vi "Lecture ParamStack.vi"(8 "errin":errorcluster, 11 "varriante":string) -> (0 "error out":errorcluster caption="errout")   [LabVIEW 2020]
uses:
  <vilib>/Utility/config.llb/Read Key (Double).vi
  <vilib>/Utility/config.llb/Read Key (String).vi
  Param_Stack.vi
  <vilib>/Utility/config.llb/NI_LVConfig.lvlib
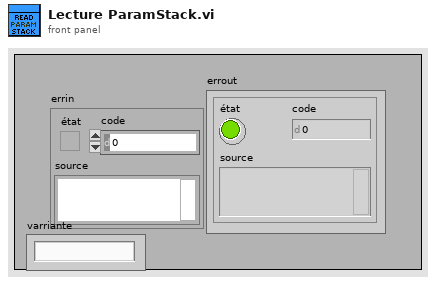
[diagram p1: front panel]
types:
  T1 = typedef "NI_LVConfig.lvlib/Config Data RefNum.ctl" = refnum<k1>
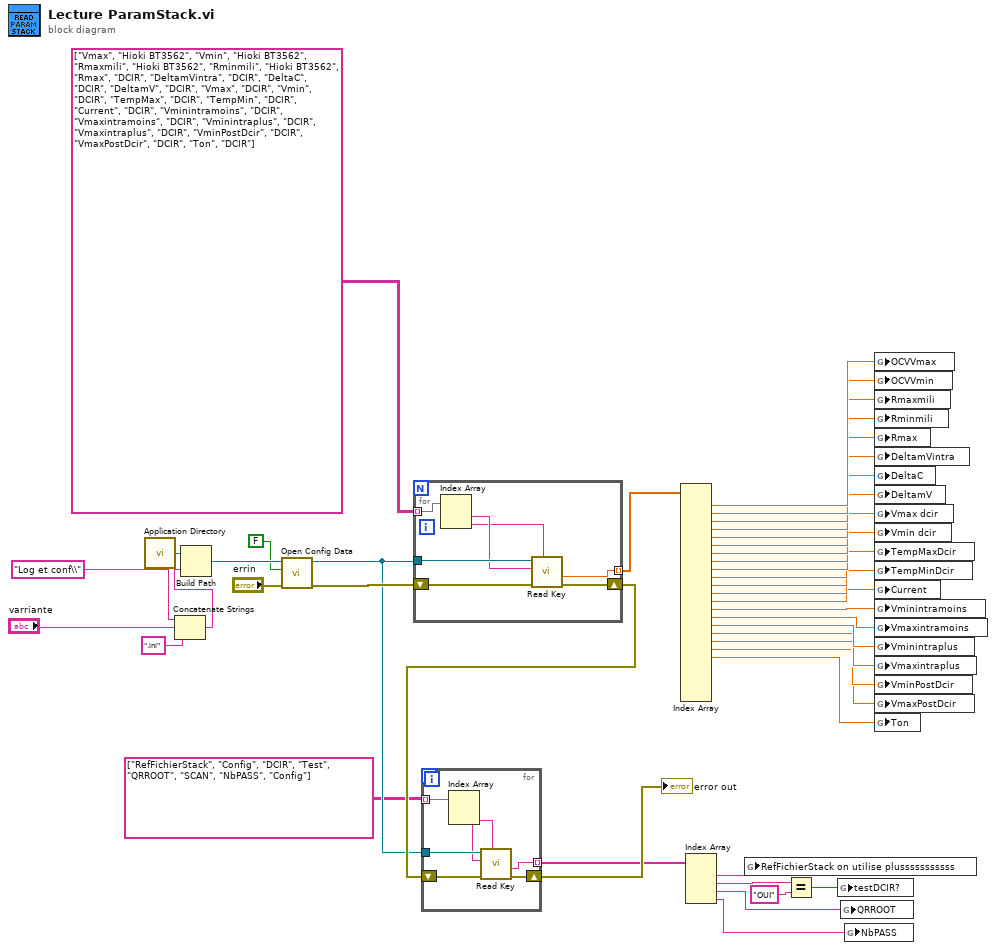
[diagram p0: block diagram]
diagram:
  n1 = call <vilib>:"Application Directory.vi"() -> ("Application Directory"=w37:path)
  n2 = Concatenate Strings("Log et conf\\", "varriante", ".ini" ("string")) -> (w4:string)
  n3 = Build Path(base path=w37, name or relative path=w4) -> (appended path=w42:path)
  n4 = call <vilib>:"Open Config Data.vi"("error in (no error)"="errin", "create file if necessary (T)"=FALSE, "configuration file path"=w42) -> ("error out"=w40:errorcluster, "refnum"=w34:T1)  [unwired: 6 in, 1 out]
  n5 = for {
    tunnel: w34 -> [w48]
    tunnel: string[][] [["Vmax", "Hioki BT3562"], ["Vmin", "Hioki BT3562"], ["Rmaxmili", "Hioki BT3562"], ["Rminmili", "Hioki BT3562"], ["Rmax", "DCIR"], ["DeltamVintra", "DCIR"], ["DeltaC", "DCIR"], ["DeltamV", "DCIR"], ["Vmax", "DCIR"], ["Vmin", "DCIR"], ["TempMax", "DCIR"], ["TempMin", "DCIR"], ["Current", "DCIR"], ["Vminintramoins", "DCIR"], ["Vmaxintramoins", "DCIR"], ["Vminintraplus", "DCIR"], ["Vmaxintraplus", "DCIR"], ["VminPostDcir", "DCIR"], ["VmaxPostDcir", "DCIR"], ["Ton", "DCIR"]] -> [w47] mode=indexing
    shift-right: [w44] -> w36
    shift-left: w40 -> [w49]
    tunnel: [w43] -> w38 mode=indexing
    n6 = Index Array(array=w47) -> (element #1=w46:string, element #2=w45:string)  [unwired: 2 in]
    n7 = call-poly <vilib>:"Read Key.vi"("section"=w45, "error in (no error)"=w49, "key"=w46, "refnum"=w48) -> ("error out"=w44:errorcluster, "value"=w43:dbl)  [unwired: 4 in, 2 out]
  }
  n8 = for {
    tunnel: w34 -> [w55]
    tunnel: string[][] [["RefFichierStack", "Config"], ["DCIR", "Test"], ["QRROOT", "SCAN"], ["NbPASS", "Config"]] -> [w54] mode=indexing
    shift-right: [w51] -> w35
    shift-left: w36 -> [w56]
    tunnel: [w50] -> w33 mode=indexing
    n9 = Index Array(array=w54) -> (element #1=w53:string, element #2=w52:string)  [unwired: 2 in]
    n10 = call-poly <vilib>:"Read Key.vi"("section"=w52, "error in (no error)"=w56, "key"=w53, "refnum"=w55) -> ("error out"=w51:errorcluster, "value"=w50:string)  [unwired: 4 in, 2 out]
  }
  "error out" <- w35
  n11 = Index Array(array=w38) -> (element #1=w30:dbl, element #2=w29:dbl, element #3=w28:dbl, element #4=w27:dbl, element #5=w26:dbl, element #6=w25:dbl, element #7=w24:dbl, element #8=w23:dbl, element #9=w22:dbl, element #10=w21:dbl, element #11=w20:dbl, element #12=w19:dbl, element #13=w18:dbl, element #14=w17:dbl, element #15=w16:dbl, element #16=w15:dbl, element #17=w14:dbl, element #18=w13:dbl, element #19=w12:dbl, element #20=w11:dbl)  [unwired: 25 in, 5 out]
  n12 = Index Array(array=w33) -> (element #1=w6:string, element #2=w10:string, element #3=w7:string, element #4=w1:string)  [unwired: 4 in]
  n13 = global write "Param_Stack.vi" "RefFichierStack on utilise plusssssssssss"(w6) -> ()
  n14 = Equal?(x=w10, y="OUI") -> (x = y?=w8:bool)
  n15 = global write "Param_Stack.vi" "testDCIR?"(w8) -> ()
  n16 = global write "Param_Stack.vi" "QRROOT"(w7) -> ()
  n17 = global write "Param_Stack.vi" "NbPASS"(w1) -> ()
  n18 = global write "Param_Stack.vi" "OCVVmax"(w30) -> ()
  n19 = global write "Param_Stack.vi" "OCVVmin"(w29) -> ()
  n20 = global write "Param_Stack.vi" "Rmaxmili"(w28) -> ()
  n21 = global write "Param_Stack.vi" "Rminmili"(w27) -> ()
  n22 = global write "Param_Stack.vi" "Rmax"(w26) -> ()
  n23 = global write "Param_Stack.vi" "DeltamVintra"(w25) -> ()
  n24 = global write "Param_Stack.vi" "DeltaC"(w24) -> ()
  n25 = global write "Param_Stack.vi" "DeltamV"(w23) -> ()
  n26 = global write "Param_Stack.vi" "Vmax dcir"(w22) -> ()
  n27 = global write "Param_Stack.vi" "Vmin dcir"(w21) -> ()
  n28 = global write "Param_Stack.vi" "TempMaxDcir"(w20) -> ()
  n29 = global write "Param_Stack.vi" "TempMinDcir"(w19) -> ()
  n30 = global write "Param_Stack.vi" "Current"(w18) -> ()
  n31 = global write "Param_Stack.vi" "Vminintramoins"(w17) -> ()
  n32 = global write "Param_Stack.vi" "Vmaxintramoins"(w16) -> ()
  n33 = global write "Param_Stack.vi" "Vminintraplus"(w15) -> ()
  n34 = global write "Param_Stack.vi" "Vmaxintraplus"(w14) -> ()
  n35 = global write "Param_Stack.vi" "VminPostDcir"(w13) -> ()
  n36 = global write "Param_Stack.vi" "VmaxPostDcir"(w12) -> ()
  n37 = global write "Param_Stack.vi" "Ton"(w11) -> ()
